vi "JKISM++ Broadcast Status Change.vi"(0 "Status with Arguments":string, 5 "State Queue":string, 7 "Broadcast(T)":bool=TRUE) -> (6 "Remaining States":string)   [LabVIEW 2014, in "JKI State Machine++.lvlib"]
doc: "Broadcast the status change to system. The JKISM++ Module who registered the status will receive the status change.\n\n<b>Inputs:</b>\n - <b>Status with Arguments</b>: Status with arguments to publish\n - <b>State Queue(\"\")</b>: The entire state queue is wired to this input.\n - <b>Broadcast(T)</b>: Trigger for broadcast or not.\n\n<b>Outputs:</b>\n - <b>Remaining States</b>: Returns all the next states that should execute after the current state completes."
uses:
  JKI State Machine++.lvlib
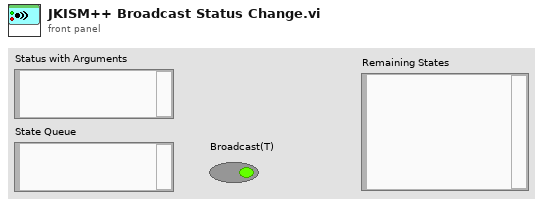
[diagram p1: front panel]
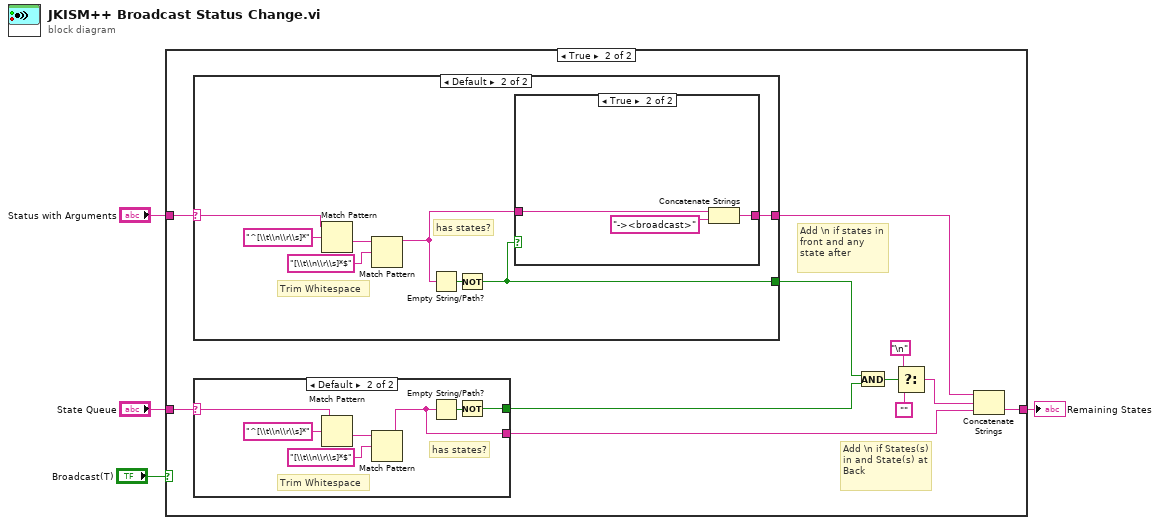
[diagram p0: block diagram]
diagram:
  n1 = case shown="True" "Broadcast(T)" {
    tunnel: [w5 w16] -> w4
    tunnel: "Status with Arguments" -> [_ w8]
    tunnel: "State Queue" -> [w5 w7]
    frame False {
    }
    frame True {
      # "Add \\n if States(s) in and State(s) at Back"
      # "Add \\n if states in front and any state after"
      n2 = case shown="Default" w8 {
        selector: w8 -> [_ w27]
        tunnel: [_ w24] -> w15
        tunnel: [_ w25] -> w10
        frame "" {
        }
        frame Default {
          # "Trim Whitespace"
          # "has states?"
          n3 = Match Pattern(string=w27, regular expression="^[\\t\\n\\r\\s]*") -> (after substring=w29:string)  [unwired: 1 in, 3 out]
          n4 = Match Pattern(string=w29, regular expression="[\\t\\n\\r\\s]*$") -> (before substring=w26:string)  [unwired: 1 in, 3 out]
          n5 = Empty String/Path?(string/path=w26) -> (empty?=w31:bool)
          n6 = Not(x=w31) -> (.not. x?=w24:bool)
          n7 = case shown="True" w24 {
            tunnel: w26 -> [w32 w35]
            tunnel: [w32 w34] -> w25
            frame False {
            }
            frame True {
              n8 = Concatenate Strings(w35, "-><broadcast>" ("string")) -> (w34:string)
            }
          }
        }
      }
      n9 = case shown="Default" w7 {
        selector: w7 -> [_ w17]
        tunnel: [_ w22] -> w6
        tunnel: [_ w18] -> w9
        frame "" {
        }
        frame Default {
          # "Trim Whitespace"
          # "has states?"
          n10 = Match Pattern(string=w17, regular expression="^[\\t\\n\\r\\s]*") -> (after substring=w20:string)  [unwired: 1 in, 3 out]
          n11 = Match Pattern(string=w20, regular expression="[\\t\\n\\r\\s]*$") -> (before substring=w18:string)  [unwired: 1 in, 3 out]
          n12 = Empty String/Path?(string/path=w18) -> (empty?=w23:bool)
          n13 = Not(x=w23) -> (.not. x?=w22:bool)
        }
      }
      n14 = And(x=w15, y=w6) -> (x .and. y?=w14:bool)
      n15 = Select(t="\n", s=w14, f="") -> (s? t:f=w13:string)
      n16 = Concatenate Strings(w10, w13, w9) -> (w16:string)
    }
  }
  "Remaining States" <- w4
